vi "Oscillation_of_MCL_Target-AidanHamilton.vi"() -> ()   [LabVIEW 2012]
uses:
  <vilib>/rvi/Emulation/niFpgaSctlEmulationGetInTimedLoop.vi
  <vilib>/rvi/Emulation/niFpgaSctlEmulationGlobalWrite.vi
  <vilib>/rvi/eio/common/nirviEmuTemplateMethod_errors.vi
  <vilib>/eio/EIONode/EIONode.xnode
panel:
  in  "Amplitude":i16
  out "Zposition MCL fine":i16
  in  "1/2 the period of oscillation":u32
  in  "Oscillation on/off":bool
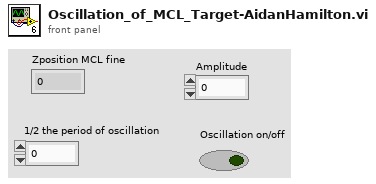
[diagram p1: front panel]
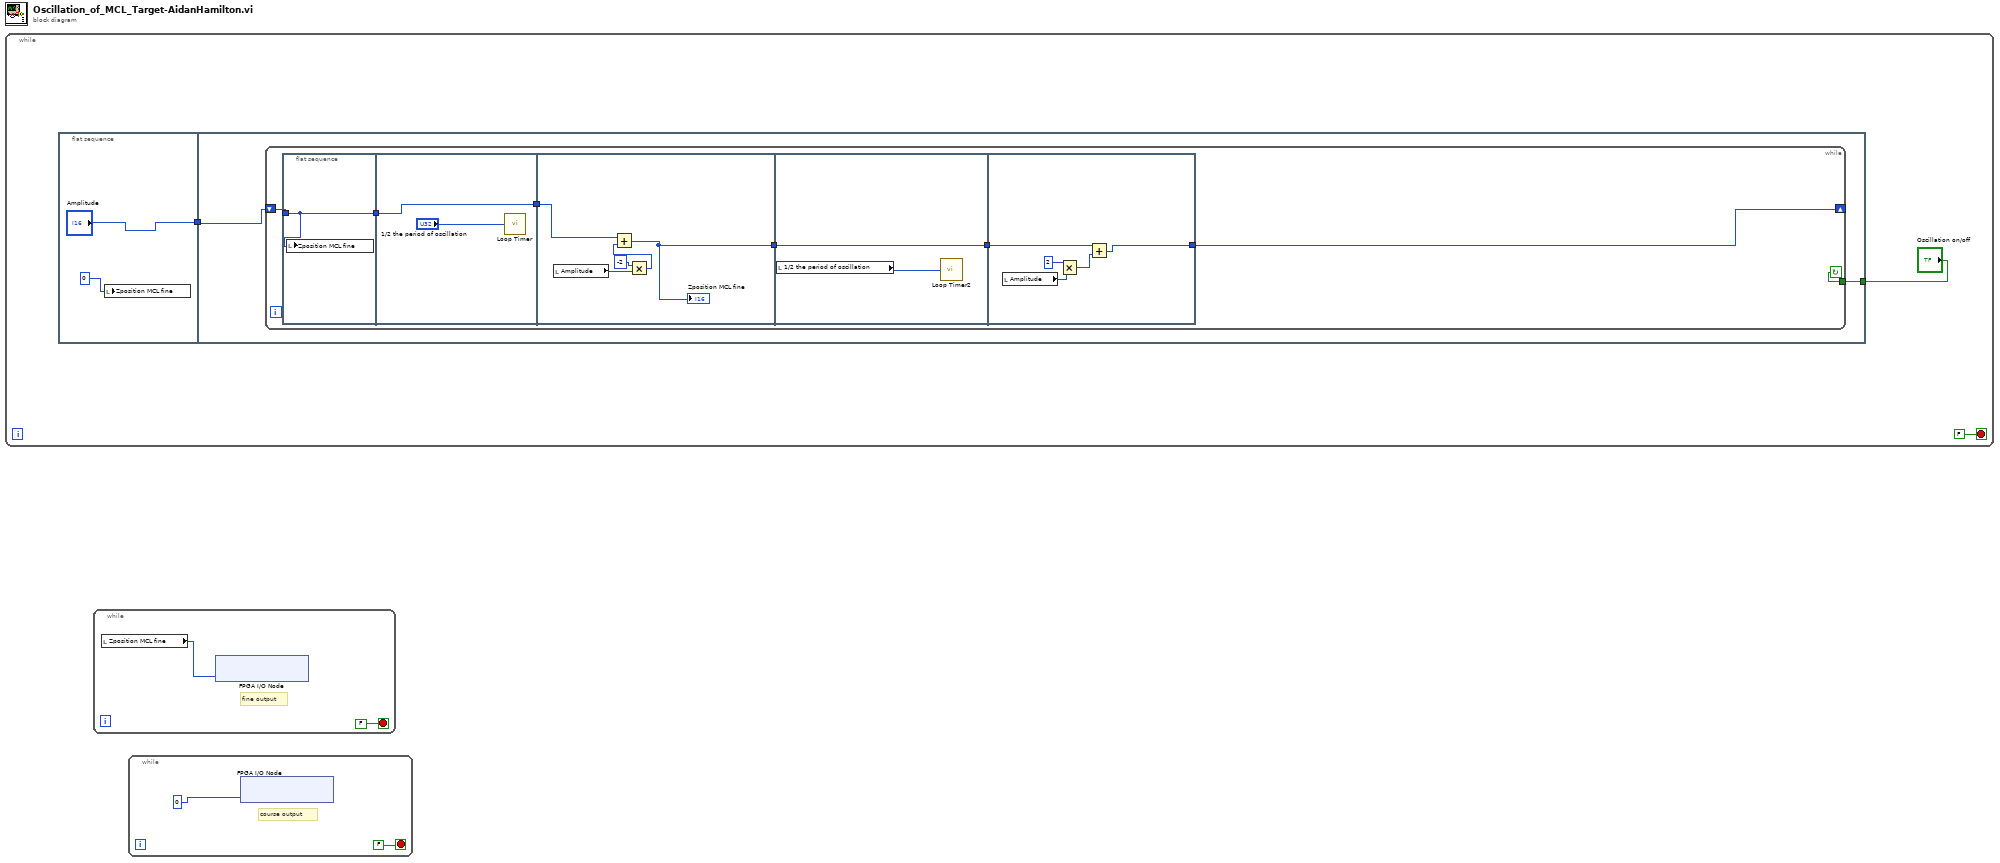
[diagram p0: block diagram]
diagram:
  n1 = while {
    stop <- FALSE stop-if-true
    n2 = flat-sequence {
      tunnel: ["Amplitude"] -> w3
      tunnel: w3 -> [w7]
      tunnel: "Oscillation on/off" -> [w6]
      frame #0 {
        n3 = local write "Zposition MCL fine"(i16 0) -> ()
      }
      frame #1 {
        n4 = while {
          shift-right: [w13] -> _
          shift-left: w7 -> [w14]
          tunnel: w6 -> [w9]
          stop <- w9 continue-if-true
          n5 = flat-sequence {
            tunnel: w14 -> [w15]
            tunnel: [w15] -> w8
            tunnel: [w16] -> w10
            tunnel: w8 -> [w16]
            tunnel: [w21] -> w12
            tunnel: w10 -> [w22]
            tunnel: w12 -> [w24]
            tunnel: [w24] -> w11
            tunnel: w11 -> [w26]
            tunnel: [w25] -> w13
            frame #0 {
              n6 = local write "Zposition MCL fine"(w15) -> ()
            }
            frame #1 {
              n7 = call "Loop Timer"("Count(uSec)"="1/2 the period of oscillation") -> ()  [unwired: 1 out]
            }
            frame #2 {
              n8 = local read "Amplitude"() -> (w20:i16)
              n9 = Multiply(x=i16 -2, y=w20) -> (x*y=w19:i16)
              n10 = Add(x=w22, y=w19) -> (x+y=w21:i16)
              "Zposition MCL fine" <- w21
            }
            frame #3 {
              n11 = local read "1/2 the period of oscillation"() -> (w23:u32)
              n12 = call "Loop Timer2"("Count(uSec)"=w23) -> ()  [unwired: 1 out]
            }
            frame #4 {
              n13 = local read "Amplitude"() -> (w27:i16)
              n14 = Multiply(x=i16 2, y=w27) -> (x*y=w29:i16)
              n15 = Add(x=w26, y=w29) -> (x+y=w25:i16)
            }
          }
        }
      }
    }
  }
  n16 = while {
    stop <- FALSE stop-if-true
    # "fine output"
    n17 = local read "Zposition MCL fine"() -> (w31:i16)
    n18 = xnode "FPGA I/O Node"("Connector0/AO7"=w31) -> ()  [unwired: 1 in, 1 out]
  }
  n19 = while {
    stop <- FALSE stop-if-true
    # "course output"
    n20 = xnode "FPGA I/O Node"("Connector0/AO2"=i16 0) -> ()  [unwired: 1 in, 1 out]
  }
